vi "calc_deltaF.vi"(8 "valid in":bool, 10 "Q in":fxp<+/-,16,14>, 11 "I in":fxp<+/-,16,14>) -> (0 "output valid":bool, 1 "delta_F":fxp<+/-,32,30>, 2 "Q out":fxp<+/-,16,14>, 3 "I out":fxp<+/-,16,14>)   [LabVIEW 2013]
uses:
  <vilib>/rvi/FXPMathLib/FxpDiv/subVIs/nifxpmath_Div_SimConfig.ctl
  <vilib>/rvi/FXPMathLib/FxpDiv/simVIs/DllFxpDivTemp_sub.vi
  <vilib>/rvi/FXPMathLib/FxpDiv/XNode/nifxpmath_Div.xnode
  <vilib>/rvi/FXPMathLib/FxpSub/XNode/nifxpmath_Sub.xnode
  <vilib>/rvi/FXPMathLib/FxpAdd/XNode/nifxpmath_Add.xnode
  <vilib>/rvi/FXPMathLib/FxpMul/XNode/nifxpmath_Multiplier.xnode
  <vilib>/rvi/FXPMathLib/sim/FxpSim.dll
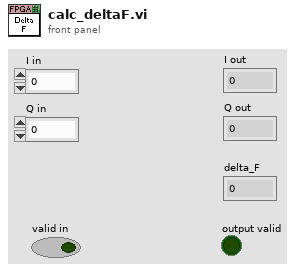
[diagram p1: front panel]
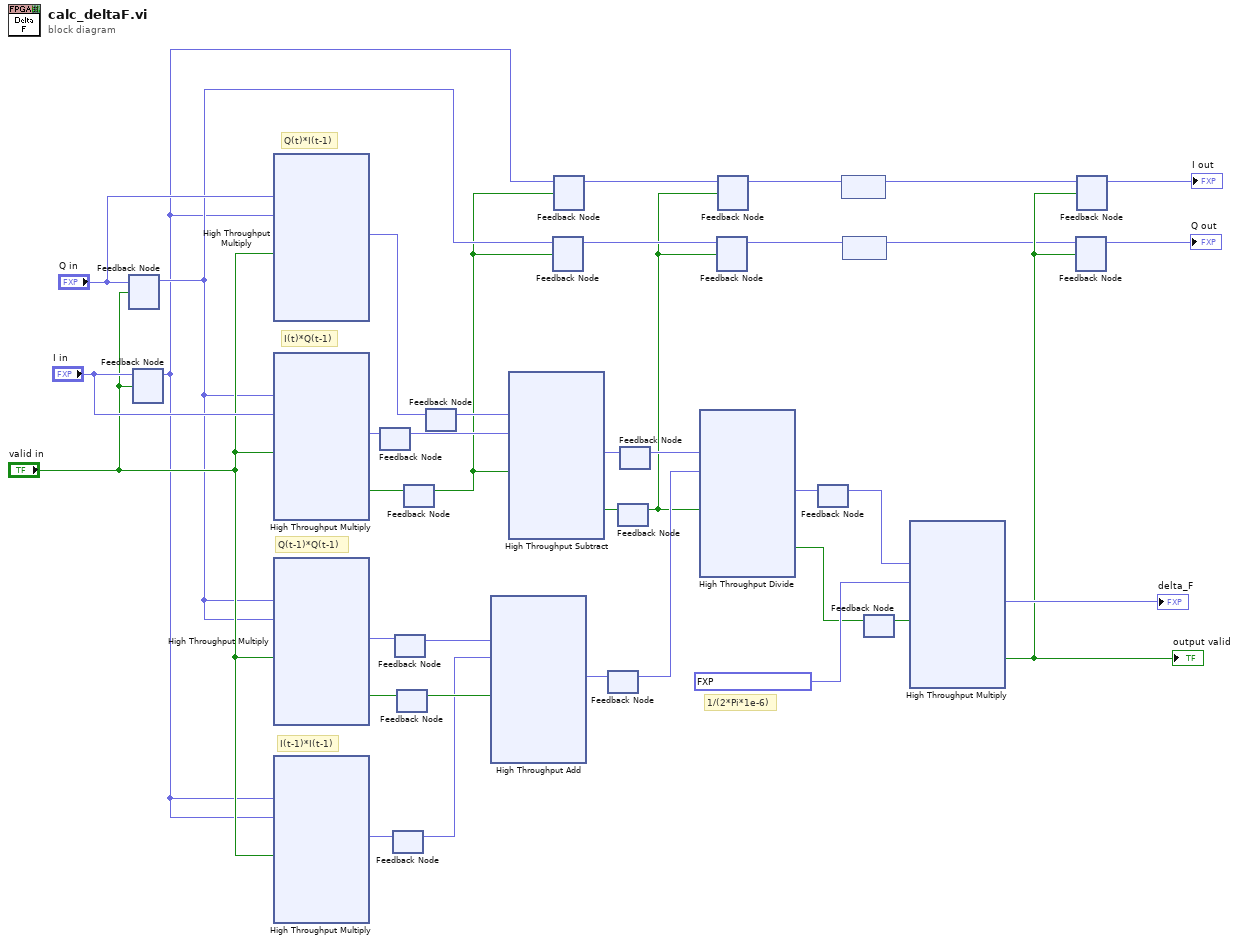
[diagram p0: block diagram]
diagram:
  # "1/(2*Pi*1e-6)"
  # "Q(t-1)*Q(t-1)"
  # "I(t-1)*I(t-1)"
  # "I(t)*Q(t-1)"
  # "Q(t)*I(t-1)"
  n1 = feedback #1() -> (w35:fxp<+/-,16,14>)  [unwired: 1 in]
  n2 = feedback-in #1("Q in", "valid in") -> ()
  n3 = feedback #2() -> (w31:fxp<+/-,16,14>)  [unwired: 1 in]
  n4 = feedback-in #2("I in", "valid in") -> ()
  n5 = xnode "High Throughput Multiply"("x"="Q in", "y"=w31, "input valid"="valid in") -> ("x*y"=w24:fxp<+/-,32,28>)  [unwired: 1 in, 2 out]
  n6 = xnode "High Throughput Multiply"("x"=w35, "y"="I in", "input valid"="valid in") -> ("x*y"=w22:fxp<+/-,32,28>, "output valid"=w20:bool)  [unwired: 1 in, 1 out]
  n7 = xnode "High Throughput Multiply"("x"=w35, "y"=w35, "input valid"="valid in") -> ("x*y"=w19:fxp<+/-,32,28>, "output valid"=w17:bool)  [unwired: 1 in, 1 out]
  n8 = xnode "High Throughput Multiply"("x"=w31, "y"=w31, "input valid"="valid in") -> ("x*y"=w15:fxp<+/-,32,28>)  [unwired: 1 in, 2 out]
  n9 = feedback #3() -> (w21:fxp<+/-,32,28>)  [unwired: 1 in]
  n10 = feedback-in #3(w22) -> ()
  n11 = feedback #4() -> (w14:fxp<+/-,32,28>)  [unwired: 1 in]
  n12 = feedback-in #4(w15) -> ()
  n13 = feedback #5() -> (w18:fxp<+/-,32,28>)  [unwired: 1 in]
  n14 = feedback-in #5(w19) -> ()
  n15 = feedback #6() -> (w16:bool)  [unwired: 1 in]
  n16 = feedback-in #6(w17) -> ()
  n17 = feedback #7() -> (w1:bool)  [unwired: 1 in]
  n18 = feedback-in #7(w20) -> ()
  n19 = feedback #8() -> (w23:fxp<+/-,32,28>)  [unwired: 1 in]
  n20 = feedback-in #8(w24) -> ()
  n21 = xnode "High Throughput Add"("x"=w18, "y"=w14, "input valid"=w16) -> ("x+y"=w11:fxp<+/-,32,29>)  [unwired: 1 in, 2 out]
  n22 = xnode "High Throughput Subtract"("x"=w23, "y"=w21, "input valid"=w1) -> ("x-y"=w13:fxp<+/-,32,29>, "output valid"=w3:bool)  [unwired: 1 in, 1 out]
  n23 = feedback #9() -> (w34:fxp<+/-,16,14>)  [unwired: 1 in]
  n24 = feedback-in #9(w35, w1) -> ()
  n25 = feedback #10() -> (w32:fxp<+/-,16,14>)  [unwired: 1 in]
  n26 = feedback-in #10(w31, w1) -> ()
  n27 = feedback #11() -> (w10:fxp<+/-,32,29>)  [unwired: 1 in]
  n28 = feedback-in #11(w11) -> ()
  n29 = feedback #12() -> (w2:bool)  [unwired: 1 in]
  n30 = feedback-in #12(w3) -> ()
  n31 = feedback #13() -> (w12:fxp<+/-,32,29>)  [unwired: 1 in]
  n32 = feedback-in #13(w13) -> ()
  n33 = xnode "High Throughput Divide"("x"=w12, "y"=w10, "input valid"=w2) -> ("x/y"=w9:fxp<+/-,32,16>, "output valid"=w7:bool)  [unwired: 1 in, 1 out]
  n34 = feedback #14() -> (w33:fxp<+/-,16,14>)  [unwired: 1 in]
  n35 = feedback-in #14(w34, w2) -> ()
  n36 = feedback #15() -> (w26:fxp<+/-,16,14>)  [unwired: 1 in]
  n37 = feedback-in #15(w32, w2) -> ()
  n38 = feedback #16() -> (w8:fxp<+/-,32,16>)  [unwired: 1 in]
  n39 = feedback-in #16(w9) -> ()
  n40 = feedback #17() -> (w25:fxp<+/-,16,14>)  [unwired: 1 in]
  n41 = feedback-in #17(w26) -> ()
  n42 = feedback #18() -> (w5:fxp<+/-,16,14>)  [unwired: 1 in]
  n43 = feedback-in #18(w33) -> ()
  n44 = feedback #19() -> (w6:bool)  [unwired: 1 in]
  n45 = feedback-in #19(w7) -> ()
  n46 = xnode "High Throughput Multiply"("x"=w8, "y"=fxp<+/-,32,20> 159154.94311523438 ("x/y"), "input valid"=w6) -> ("x*y"=→"delta_F":fxp<+/-,32,30>, "output valid"=w28:bool)  [unwired: 1 in, 1 out]
  "output valid" <- w28
  n47 = feedback #20() -> (→"Q out":fxp<+/-,16,14>)  [unwired: 1 in]
  n48 = feedback-in #20(w5, w28) -> ()
  n49 = feedback #21() -> (→"I out":fxp<+/-,16,14>)  [unwired: 1 in]
  n50 = feedback-in #21(w25, w28) -> ()
